vi "配置Bark UI.vi"() -> ()   [LabVIEW 2016]
panel:
  in  "Test":bool
  in  "保存":bool
  in  "url 3":string
  in  "url 2":string
  in  "url":string
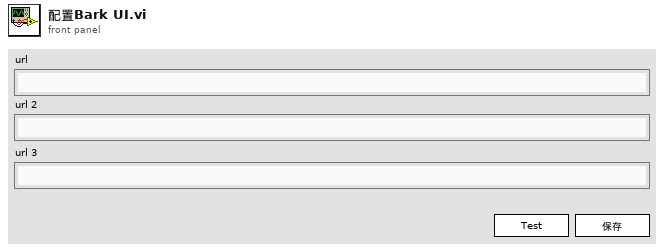
[diagram p1: front panel]
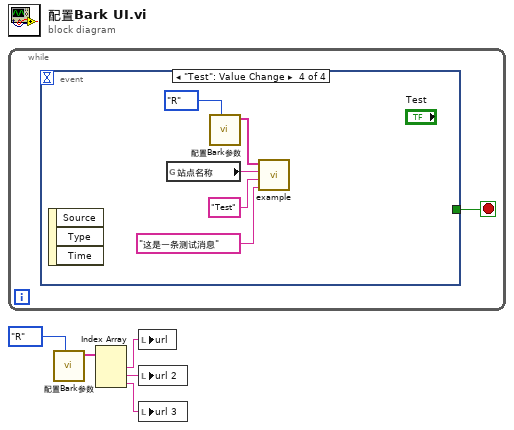
[diagram p0: block diagram]
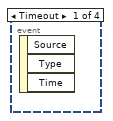
[diagram p2: hidden frame]
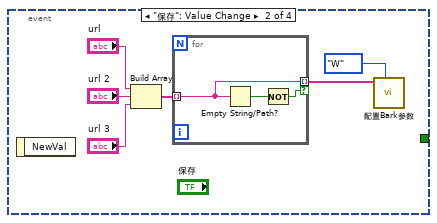
[diagram p3: hidden frame]
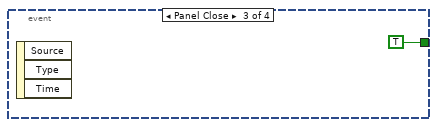
[diagram p4: hidden frame]
diagram:
  n1 = while {
    stop <- w6 stop-if-true
    n2 = event shown="[3] \"Test\": Value Change" {
      selector: _ -> [_ _ _ _]
      dyn-events: _ -> [_ _ _ _]
      timeout: _ -> [_ _ _ _]
      tunnel: [_ _ TRUE _] -> w6
      event Timeout {
        n3 = event-data() -> ()  [unwired: 1 in, 3 out]
      }
      event "保存": Value Change {
        n4 = event-data() -> ()  [unwired: 1 in, 1 out]
        n5 = Build Array("url", "url 2", "url 3") -> (w9:string[])
        n6 = for {
          tunnel: w9 -> [w14] mode=indexing
          tunnel: [w14] -> w8 mode=indexing if=w13
          n7 = Empty String/Path?(string/path=w14) -> (empty?=w15:bool)
          n8 = Not(x=w15) -> (.not. x?=w13:bool)
        }
        n9 = call "配置Bark参数.vi"("FUN"=enum16{"W", "R"}."W", "URLs"=w8) -> ()  [unwired: 9 in, 1 out]
      }
      event Panel Close {
        n10 = event-data() -> ()  [unwired: 1 in, 3 out]
      }
      event "Test": Value Change {
        n11 = event-data() -> ()  [unwired: 1 in, 3 out]
        n12 = global read "系统设置全局变量.vi" "站点名称"() -> (w19:string)
        n13 = call "配置Bark参数.vi"("FUN"=enum16{"W", "R"}."R") -> ("URLs 2"=w20:string[])  [unwired: 10 in]
        n14 = call "example.vi"("Message"="这是一条测试消息", "Title"="Test", "Group"=w19, "urls"=w20) -> ()  [unwired: 8 in]
      }
    }
  }
  n15 = call "配置Bark参数.vi"("FUN"=enum16{"W", "R"}."R") -> ("URLs 2"=w4:string[])  [unwired: 10 in]
  n16 = Index Array(array=w4) -> (element #1=w3:string, element #2=w2:string, element #3=w1:string)  [unwired: 3 in]
  n17 = local write "url"(w3) -> ()
  n18 = local write "url 2"(w2) -> ()
  n19 = local write "url 3"(w1) -> ()
